vi "Start continuous acquisition.vi"(5 "N-samples":i32, 6 "Timeout":i32=-1, 7 "Average?":bool, 8 "error in":errorcluster, 10 "Parameter":u16(ring)=1 items=["X"=1, "Y"=2, "R"=3, "Theta"=4, "Channel 1"=5, "Channel 2"=6, "Aux In 1"=7, "Aux In 2"=8, "Aux In 3"=9, "Aux In 4"=10], 11 "Module ID":i32=-1) -> (0 "error out":errorcluster)   [LabVIEW 2020, in "Lock-in amplifier.lvlib"]
doc: "Request to acquire continuously and return a single sample or an average of samples.\n_____\nCreated using DQMH Event Scripter 6.1.0.128."
uses:
  Lock-in amplifier.lvlib
  Start continuous acquisition Argument--cluster.ctl
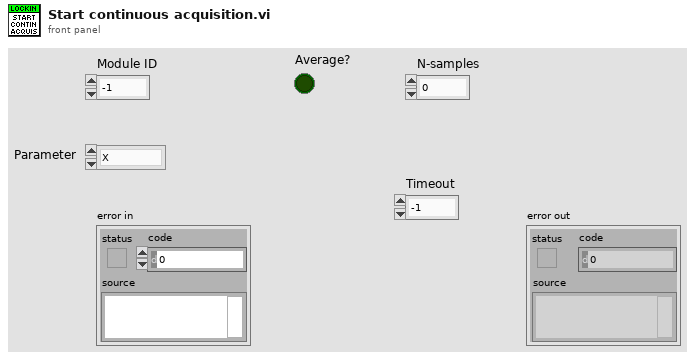
[diagram p1: front panel]
types:
  T1 = typedef "Lock-in amplifier.lvlib/Start continuous acquisition Argument--cluster.ctl" = cluster{"Module ID":i32, "Average?":bool, "N-samples":i32, "Parameter":u16, "Timeout":i32}
  T2 = typedef "Lock-in amplifier.lvlib/Request Events--cluster.ctl" = cluster{"Stop Module":refnum<user-event>, "Show Panel":refnum<user-event>, "Hide Panel":refnum<user-event>, "Show Diagram":refnum<user-event>, "Get Module Execution Status":refnum<user-event>, "Draw Panel into Subpanel":refnum<user-event>, "Remove Panel from Subpanel":refnum<user-event>, "Connect":refnum<user-event>, "Read datapoint":refnum<user-event>, "Average samples":refnum<user-event>, "Disconnect":refnum<user-event>, "Configure":refnum<user-event>, "Start continuous acquisition":refnum<user-event>, "Stop continuous acquisition":refnum<user-event>}
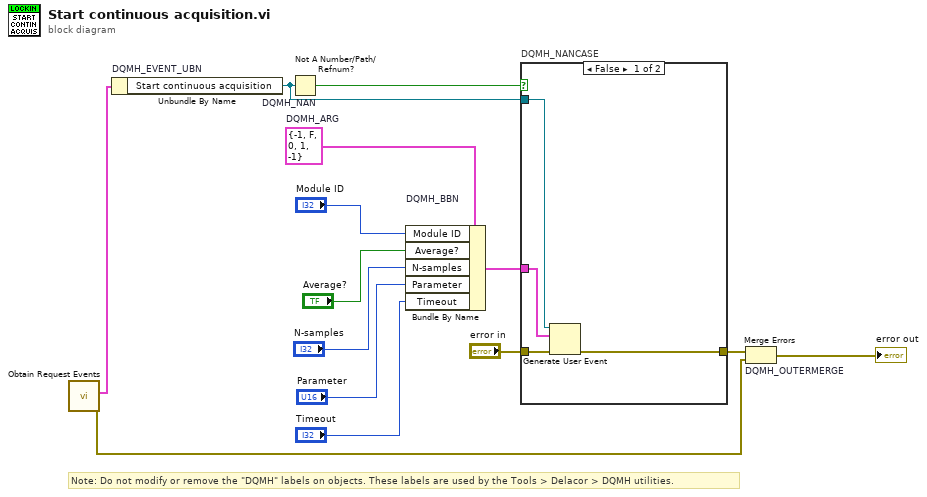
[diagram p0: block diagram]
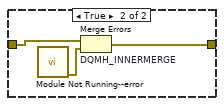
[diagram p2: hidden frame]
diagram:
  w8 = T1 {"Module ID"=-1, "Average?"=FALSE, "N-samples"=0, "Parameter"=1, "Timeout"=-1}  # DQMH_ARG
  # "Note: Do not modify or remove the \"DQMH\" labels on objects. These labels are used by the Tools > Delacor > DQMH utilities."
  n1 = call "Obtain Request Events.vi"() -> ("error out"=w3:errorcluster, "Lock-in amplifier Request Events"=w2:T2)  [unwired: 10 in]
  n2 = Unbundle By Name "DQMH_EVENT_UBN"(w2) -> ("Start continuous acquisition"=w10:refnum<user-event>)
  n3 = Not A Number/Path/Refnum? "DQMH_NAN"(number/path/refnum=w10) -> (NaN/Path/Refnum?=w11:bool)
  n4 = Bundle By Name "DQMH_BBN"(cluster=w8, "Module ID"="Module ID", "Average?"="Average?", "N-samples"="N-samples", "Parameter"="Parameter", "Timeout"="Timeout") -> (w12:T1)
  n5 = case "DQMH_NANCASE" shown="False" w11 {
    tunnel: "error in" -> [w18 w21]
    tunnel: [w17 w20] -> w9
    tunnel: w10 -> [w16 _]
    tunnel: w12 -> [w15 _]
    frame False {
      n6 = Generate User Event(user event=w16, event data cluster=w15, error in=w18) -> (error out=w17:errorcluster)  [unwired: 1 in, 1 out]
    }
    frame True {
      n7 = call "Module Not Running--error.vi"() -> ("error out"=w19:errorcluster)  [unwired: 11 in]
      n8 = Merge Errors "DQMH_INNERMERGE"(w21, w19) -> (w20:errorcluster)
    }
  }
  n9 = Merge Errors "DQMH_OUTERMERGE"(w9, w3) -> (→"error out":errorcluster)
